vi "transmitData.vi"(8 "error in (no error)":errorcluster, 10 "Data":u8[](array[numeric]), 11 "TCP Network Connection in":refnum<k5>) -> (0 "error out":errorcluster, 3 "TCP Network Connection out":refnum<k5>)   [LabVIEW 2014]
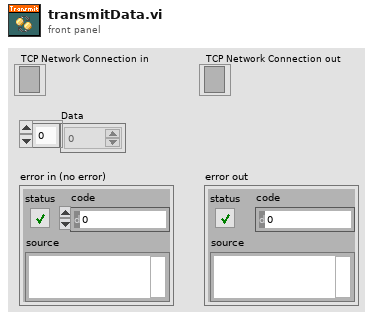
[diagram p1: front panel]
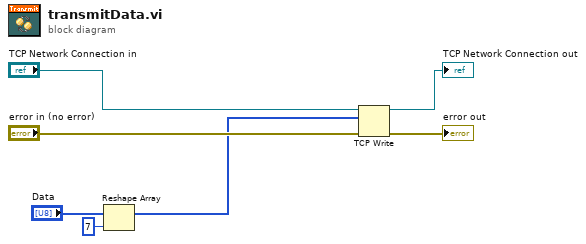
[diagram p0: block diagram]
diagram:
  n1 = Reshape Array("Data", 7 ("dimension size")) -> (w2:u8[])
  n2 = TCP Write(connection ID="TCP Network Connection in", data in=w2, error in (no error)="error in (no error)") -> (connection ID out=→"TCP Network Connection out":refnum<k5>, error out=→"error out":errorcluster)  [unwired: 1 in, 1 out]
